vi "RichToFlatnidaqmx_grpc_GetTaskAttributeStringRequest.vi"(5 "OutputClusterType":T1, 11 "InputCluster":T4) -> (3 "OutputCluster":T1)   [LabVIEW 2021, in "NI_DAQmx_client.lvlib"]
uses:
  NI_DAQmx_client.lvlib
  nidaqmx_grpc_GetTaskAttributeStringRequest.ctl
  nidevice_grpc_Session_session/nidevice_grpc_Session_session.lvclass
  nidaqmx_grpc_GetTaskAttributeStringRequest_attribute_enum/nidaqmx_grpc_GetTaskAttributeStringRequest_attribute_enum.lvclass
  nidevice_grpc_Session.ctl
  nidaqmx_grpc_GetTaskAttributeStringRequest_Flat.ctl
  nidevice_grpc_Session_Flat.ctl
  nidaqmx_grpc_TaskStringAttribute.ctl
  nidevice_grpc_Session_session/nidevice_grpc_Session_session.lvclass/nidevice_grpc_Session_session.ctl
  nidaqmx_grpc_GetTaskAttributeStringRequest_attribute_enum/nidaqmx_grpc_GetTaskAttributeStringRequest_attribute_enum.lvclass/nidaqmx_grpc_GetTaskAttributeStringRequest_attribute_enum.ctl
  nidevice_grpc_Session_session/Getname.vi
  nidevice_grpc_Session_session/Getid.vi
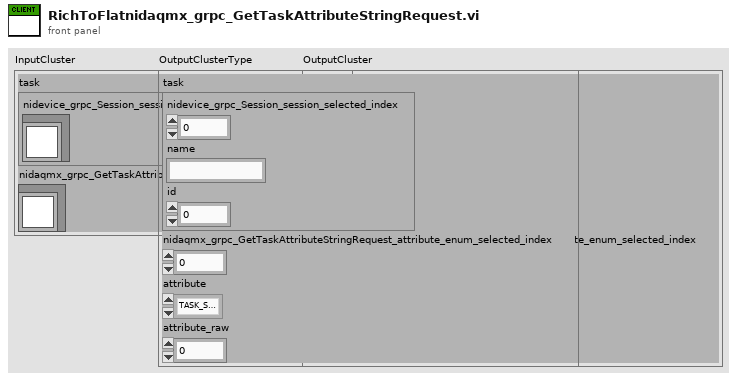
[diagram p1: front panel]
types:
  T1 = typedef "NI_DAQmx_client.lvlib/nidaqmx_grpc_GetTaskAttributeStringRequest_Flat.ctl" = cluster{"task":T2, "nidaqmx_grpc_GetTaskAttributeStringRequest_attribute_enum_selected_index":i32, "attribute":T3, "attribute_raw":i32}
  T2 = typedef "NI_DAQmx_client.lvlib/nidevice_grpc_Session_Flat.ctl" = cluster{"nidevice_grpc_Session_session_selected_index":i32, "name":string, "id":u32}
  T3 = typedef "NI_DAQmx_client.lvlib/nidaqmx_grpc_TaskStringAttribute.ctl" = enum32{"TASK_STRING_ATTRIBUTE_UNSPECIFIED", "TASK_ATTRIBUTE_CHANNELS", "TASK_ATTRIBUTE_NAME", "TASK_ATTRIBUTE_DEVICES"}
  T4 = typedef "NI_DAQmx_client.lvlib/nidaqmx_grpc_GetTaskAttributeStringRequest.ctl" = cluster{"task":T5, "nidaqmx_grpc_GetTaskAttributeStringRequest_attribute_enum":refnum<class "nidaqmx_grpc_GetTaskAttributeStringRequest_attribute_enum.lvclass">}
  T5 = typedef "NI_DAQmx_client.lvlib/nidevice_grpc_Session.ctl" = cluster{"nidevice_grpc_Session_session":refnum<class "nidevice_grpc_Session_session.lvclass">}
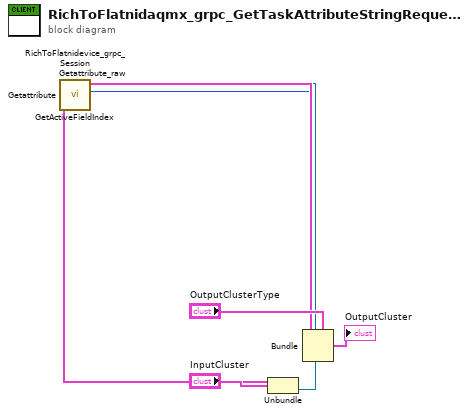
[diagram p0: block diagram]
diagram:
  n1 = Unbundle "Unbundle"("InputCluster") -> ("task"=w6:T5, "nidaqmx_grpc_GetTaskAttributeStringRequest_attribute_enum"=w4:refnum<class "nidaqmx_grpc_GetTaskAttributeStringRequest_attribute_enum.lvclass">)
  n2 = call "Getattribute_raw.vi"("OneOfTemplate in"=w4) -> ("Get_Val"=w1:i32)  [unwired: 8 in, 2 out]
  n3 = call "Getattribute.vi"("OneOfTemplate in"=w4) -> ("Get_Val"=w2:T3)  [unwired: 8 in, 2 out]
  n4 = call "GetActiveFieldIndex.vi"("OneOfTemplate in"=w4) -> ("Active Field Index"=w3:i32)  [unwired: 8 in, 2 out]
  n5 = call "RichToFlatnidevice_grpc_Session.vi"("InputCluster"=w6) -> ("OutputCluster"=w5:T2)  [unwired: 10 in]
  n6 = Bundle "Bundle"(cluster="OutputClusterType", "task"=w5, "nidaqmx_grpc_GetTaskAttributeStringRequest_attribute_enum_selected_index"=w3, "attribute"=w2, "attribute_raw"=w1) -> (→"OutputCluster":T1)
